vi "Write Loop.vi"(8 "error in (no error)":errorcluster, 11 "WAMP Client in":refnum<class "WAMP Client.lvclass">) -> (0 "error out":errorcluster, 3 "WAMP Client out":refnum<class "WAMP Client.lvclass">)   [LabVIEW 2020, in "wamplv.lvlib" / "WAMP Client.lvclass"]
uses:
  <vilib>/samangh/wamplv/WAMP Client/WAMP Client.lvclass
  <vilib>/samangh/wamplv/WAMP Client/WAMP Client.lvclass/WAMP Client.ctl
  <vilib>/samangh/wamplv/WAMP Client/TypeDef/Termination Reason Enum.ctl
  <vilib>/samangh/wamplv/Comm Handlers/ICommHandler/ICommHandler.lvclass
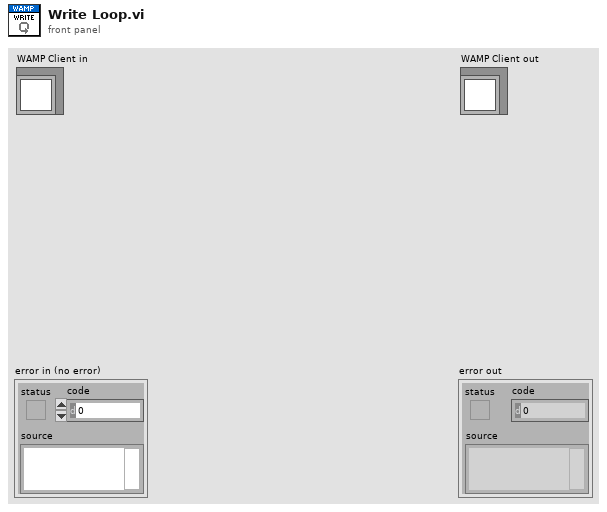
[diagram p1: front panel]
types:
  T1 = typedef "wamplv.lvlib/WAMP Client.lvclass/Termination Reason Enum.ctl" = enum16{"Goodbye Received", "Abort Received", "Send Goodbye", "Send Abort", "Read Loop Failure", "Write Loop Failure", "Message Loop Failure"}
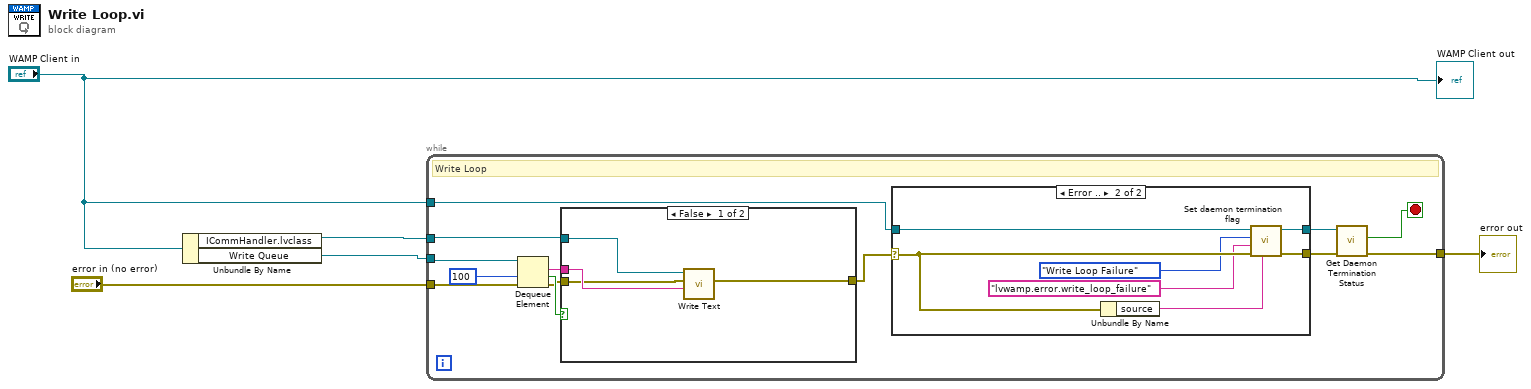
[diagram p0: block diagram]
diagram:
  n1 = Unbundle By Name("WAMP Client in") -> ("ICommHandler.lvclass"=w5:refnum<class "ICommHandler.lvclass">, "Write Queue"=w4:refnum<queue>)
  n2 = while {
    tunnel: w4 -> [w18]
    tunnel: w5 -> [w17]
    tunnel: "error in (no error)" -> [w12]
    tunnel: [w7] -> w2
    tunnel: "WAMP Client in" -> [w6]
    stop <- w8 stop-if-true
    # "Write Loop"
    n3 = Dequeue Element(queue=w18, timeout in ms (-1)=100, error in (no error)=w12) -> (element=w16:string, timed out?=w15:bool, error out=w14:errorcluster)  [unwired: 1 out]
    n4 = case shown="False" w15 {
      tunnel: w17 -> [w31 _]
      tunnel: w16 -> [w30 _]
      tunnel: w14 -> [w29 w32]
      tunnel: [w28 w32] -> w11
      frame False {
        n5 = call-dynamic "Write Text.vi"("String"=w30, "error in (no error)"=w29, "ICommHandler in"=w31) -> ("error out"=w28:errorcluster)  [unwired: 7 in, 1 out]
      }
      frame True {
        # "Queue is empty, do nothing"
      }
    }
    n6 = case shown="Error .." w11 {
      selector: w11 -> [w20 w26]
      tunnel: [w20 w27] -> w10
      tunnel: [w19 w25] -> w9
      tunnel: w6 -> [w19 w21]
      frame No Error {
      }
      frame Error {
        n7 = Unbundle By Name(w26) -> ("source"=w22:string)
        n8 = call <vilib>:"Set daemon termination flag.vi"("Message"=w22, "error in (no error)"=w26, "Reason URI"="lvwamp.error.write_loop_failure" ("Error URI"), "Reason"=Termination_Reason_Enum."Write Loop Failure" ("Termination Reason"), "WAMP Client (in)"=w21) -> ("error out"=w27:errorcluster, "WAMP Client (out)"=w25:refnum<class "WAMP Client.lvclass">)  [unwired: 5 in]
      }
    }
    n9 = call <vilib>:"Get Daemon Termination Status.vi"("error in (no error)"=w10, "WAMP Client in"=w9) -> ("error out"=w7:errorcluster, "Terminate?"=w8:bool)  [unwired: 6 in, 2 out]
  }
  "error out" <- w2
  "WAMP Client out" <- "WAMP Client in"
